vi "Write RIO Device.vi"(8 "error in (no error)":errorcluster, 10 "RIO Device":T1, 11 "FPGA Module configuration in":refnum<class "FPGA Module configuration.lvclass">) -> (0 "error out":errorcluster, 3 "FPGA Module configuration out":refnum<class "FPGA Module configuration.lvclass">)   [LabVIEW 2014, in "FPGA Module configuration.lvclass"]
uses:
  FPGA Module configuration.lvclass
  <vilib>/userdefined/High Color/nirio_resource_hc.ctl
  FPGA Module configuration.lvclass/FPGA Module configuration.ctl
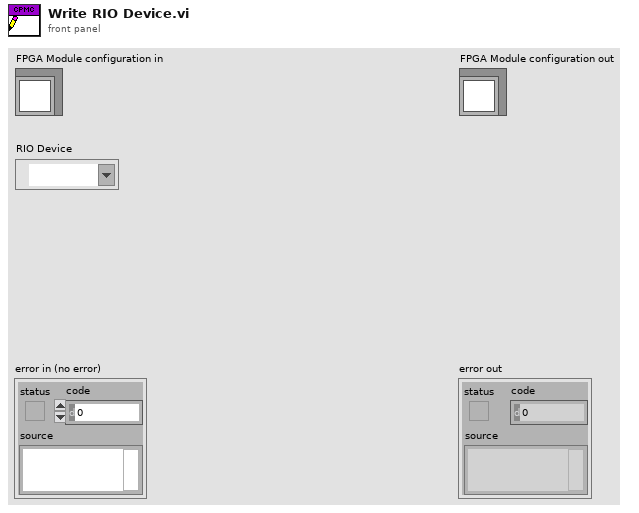
[diagram p1: front panel]
types:
  T1 = typedef "nirio_resource_hc.ctl" = tag
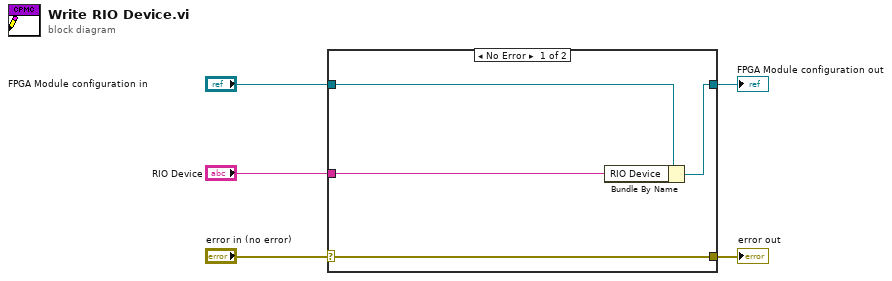
[diagram p0: block diagram]
diagram:
  n1 = case shown="No Error" "error in (no error)" {
    selector: "error in (no error)" -> [w9 w10]
    tunnel: [w9 w10] -> w4
    tunnel: [w7 w11] -> w2
    tunnel: "FPGA Module configuration in" -> [w8 w11]
    tunnel: "RIO Device" -> [w6 _]
    frame No Error {
      n2 = Bundle By Name(cluster=w8, "RIO Device"=w6) -> (w7:refnum<class "FPGA Module configuration.lvclass">)
    }
    frame Error {
    }
  }
  "error out" <- w4
  "FPGA Module configuration out" <- w2
